vi "Run Test.vi"(8 "error in (no error)":errorcluster, 11 "Test Template in":refnum<class "LCM Single-Up MTS Test.lvclass">) -> (0 "error out":errorcluster, 1 "Fail Codes":string[](array[string]), 2 "Tests Passed":bool[](array[boolean]), 3 "Test Template out":refnum<class "LCM Single-Up MTS Test.lvclass">)   [LabVIEW 2015, in "LCM Single-Up MTS Test.lvclass"]
uses:
  LCM Single-Up MTS Test.lvclass
  Test Class/Test Class.lvclass/Test Class.ctl
  Test Class/Test Class.lvclass
  Classes/Application/Class/Application.lvclass
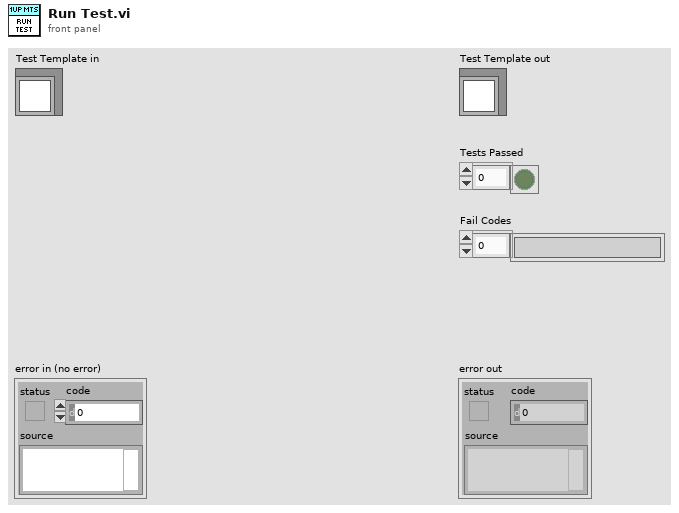
[diagram p1: front panel]
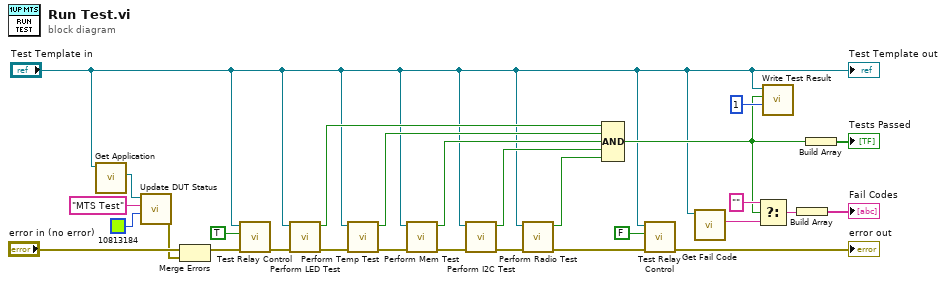
[diagram p0: block diagram]
diagram:
  n1 = call "Get Application.vi"("Test Class in"="Test Template in") -> ("Application.lvlib:Application.lvclass"=w18:refnum<class "Application.lvclass">)  [unwired: 9 in, 1 out]
  n2 = call "Update DUT Status.vi"("BG Color"=u32 10813184, "Message ('')"="MTS Test", "Application in"=w18) -> ("error out"=w14:errorcluster)  [unwired: 7 in, 1 out]
  n3 = Merge Errors("error in (no error)", w14) -> (w7:errorcluster)
  n4 = call-dynamic "Test Relay Control.vi"("error in (no error)"=w7, "Connect (False)"=TRUE, "LCM Single-Up MTS Test in"="Test Template in") -> ("error out"=w6:errorcluster)  [unwired: 8 in]
  n5 = call "Perform LED Test.vi"("error in (no error)"=w6, "LCM Single-Up MTS Test in"="Test Template in") -> ("error out"=w24:errorcluster, "LED Test Passed"=w27:bool)  [unwired: 8 in]
  n6 = call "Perform Temp Test.vi"("error in (no error)"=w24, "LCM Single-Up MTS Test in"="Test Template in") -> ("error out"=w11:errorcluster, "Temperature Test Passed"=w26:bool)  [unwired: 8 in]
  n7 = call "Perform Mem Test.vi"("error in (no error)"=w11, "LCM Single-Up MTS Test in"="Test Template in") -> ("error out"=w5:errorcluster, "Memory Test Passed"=w25:bool)  [unwired: 8 in]
  n8 = call "Perform I2C Test.vi"("error in (no error)"=w5, "LCM Single-Up MTS Test in"="Test Template in") -> ("error out"=w4:errorcluster, "I2C Data Match"=w13:bool)  [unwired: 8 in]
  n9 = call "Perform Radio Test.vi"("error in (no error)"=w4, "LCM Single-Up MTS Test in"="Test Template in") -> ("error out"=w1:errorcluster, "Radio Test Passed"=w2:bool)  [unwired: 8 in]
  n10 = Compound Arithmetic op=AND(w27, w26, w25, w13, w2) -> (w9:bool)
  n11 = call-dynamic "Test Relay Control.vi"("error in (no error)"=w1, "Connect (False)"=FALSE, "LCM Single-Up MTS Test in"="Test Template in") -> ("error out"=→"error out":errorcluster)  [unwired: 8 in]
  n12 = call "Get Fail Code.vi"("Test Class in"="Test Template in") -> ("Fail Code"=w12:string)  [unwired: 9 in, 1 out]
  n13 = Select(t="", s=w9, f=w12) -> (s? t:f=w22:string)
  n14 = call "Write Test Result.vi"("Position"=u32 1, "Test Passed"=w9, "Test Class.lvclass"="Test Template in") -> ()  [unwired: 9 in]
  n15 = Build Array(w22) -> (→"Fail Codes":string[])
  n16 = Build Array(w9) -> (→"Tests Passed":bool[])
  "Test Template out" <- "Test Template in"
